vi "ICNC Move Speed Abs Local Buf.vi"(0 "Axis":u32, 1 "MoveZ":i32, 2 "MoveB":i32, 5 "Speed":u32, 7 "MoveX":i32, 9 "MoveY":i32, 11 "error in (no error)":errorcluster caption="entrée d'erreur (pas d'erreur)", 12 "MoveA":i32, 13 "BufferRequired":u32) -> (4 "BufferRequired out":u32, 6 "function return":u32, 15 "error out":errorcluster caption="sortie d'erreur")   [LabVIEW 2012, in "ICNC2.lvlib"]
doc: "DWORD ICNC_MoveSpeedAbsLocalBuf (DWORD Axis,\n DWORD Speed,\n INT MoveX,\n INT MoveY,\n INT MoveZ,\n INT MoveA,\n INT MoveB,\n DWORD *BufferRequired=NULL);"
uses:
  <userlib>/ICNC/ICNC2.lvlib
  <userlib>/ICNC/ICNC2.dll
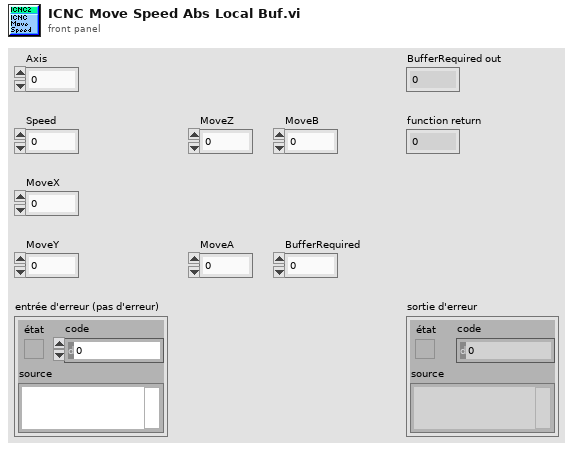
[diagram p1: front panel]
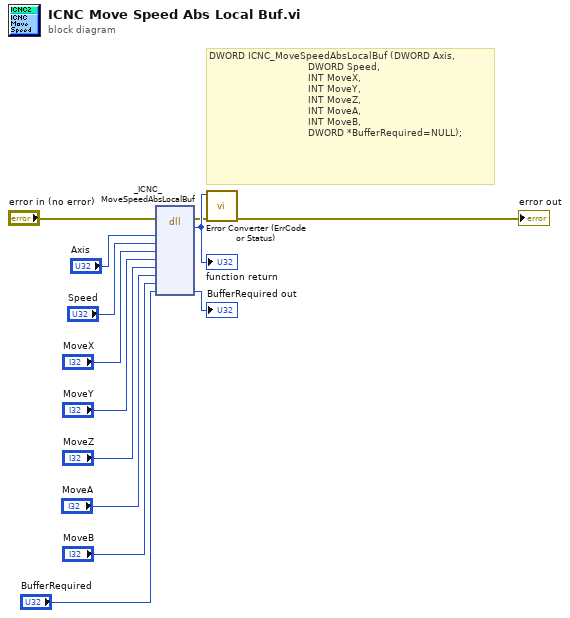
[diagram p0: block diagram]
diagram:
  # "DWORD ICNC_MoveSpeedAbsLocalBuf (DWORD Axis,\n                                 DWORD Speed,\n                                 INT MoveX,\n                                 INT MoveY,\n                                 INT MoveZ,\n                                 INT MoveA,\n                                 INT MoveB,\n                                 DWORD *BufferRequired=NULL);"
  n1 = dll-call lib="C:/Program Files (x86)/National Instruments/LabVIEW 2012/user.lib/ICNC/ICNC2.*" fn="_ICNC_MoveSpeedAbsLocalBuf"(error in="error in (no error)", "Axis"="Axis", "Speed"="Speed", "MoveX"="MoveX", "MoveY"="MoveY", "MoveZ"="MoveZ", "MoveA"="MoveA", "MoveB"="MoveB", "BufferRequired"="BufferRequired") -> (error out=w2:errorcluster, w13:u32, "BufferRequired"=→"BufferRequired out":u32)  [unwired: 9 in, 1 out]
  "function return" <- w13
  n2 = call <userlib>:"Error Converter (ErrCode or Status).vi"("error in (no error)"=w2, "error code"=w13) -> ("error out"=→"error out":errorcluster)  [unwired: 9 in]
